vi "client handle page request.vi"(4 "error in (no error)":errorcluster, 7 "Client IP (\"\")":string) -> (0 "error out":errorcluster, 3 "Template Keys":T1)   [LabVIEW 2011]
uses:
  Addons/internet/utils/keyedarr.llb/Keyed Array.ctl
  Addons/internet/utils/strutil.llb/Case Matching.ctl
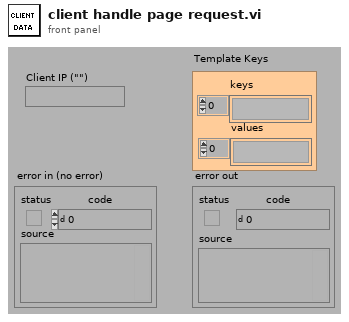
[diagram p1: front panel]
types:
  T1 = typedef "Keyed Array.ctl" = cluster{"keys":string[], "values":string[]}
  T2 = typedef "Case Matching.ctl" = enum16{"a != A", "a == A", "system"}
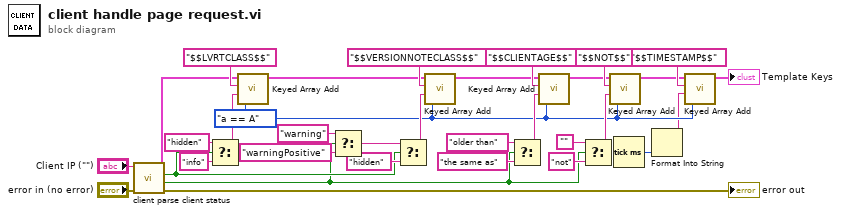
[diagram p0: block diagram]
diagram:
  w7 = Case_Matching."a == A" ("case matching (sensitive)")
  n1 = call "client parse client status.vi"("error in (no error)"="error in (no error)", "Client IP"="Client IP (\"\")") -> ("error out"=→"error out":errorcluster, "Update Needed?"=w2:bool, "Client Detected?"=w14:bool, "Client Status Keys"=w15:T1)  [unwired: 6 out]
  n2 = Select(t="hidden" ("Template (\"\")"), s=w14, f="info" ("Template (\"\")")) -> (s? t:f=w26:string)
  n3 = call "Keyed Array Add.vi"("case matching (sensitive)"=w7, "value"=w26, "key"="$$LVRTCLASS$$" ("Template (\"\")"), "array in"=w15) -> ("array out"=w31:T1)  [unwired: 3 out]
  n4 = Select(t="warning" ("Template (\"\")"), s=w2, f="warningPositive" ("Template (\"\")")) -> (s? t:f=w1:string)
  n5 = Select(t=w1, s=w14, f="hidden" ("Template (\"\")")) -> (s? t:f=w25:string)
  n6 = call "Keyed Array Add.vi"("case matching (sensitive)"=w7, "value"=w25, "key"="$$VERSIONNOTECLASS$$" ("Template (\"\")"), "array in"=w31) -> ("array out"=w29:T1)  [unwired: 3 out]
  n7 = Select(t="older than" ("Template (\"\")"), s=w2, f="the same as" ("Template (\"\")")) -> (s? t:f=w19:string)
  n8 = call "Keyed Array Add.vi"("case matching (sensitive)"=w7, "value"=w19, "key"="$$CLIENTAGE$$" ("Template (\"\")"), "array in"=w29) -> ("array out"=w27:T1)  [unwired: 3 out]
  n9 = Select(t="", s=w2, f="not" ("Template (\"\")")) -> (s? t:f=w16:string)
  n10 = call "Keyed Array Add.vi"("case matching (sensitive)"=w7, "value"=w16, "key"="$$NOT$$" ("Template (\"\")"), "array in"=w27) -> ("array out"=w9:T1)  [unwired: 3 out]
  n11 = Tick Count (ms)() -> (millisecond timer value=w6:u32)
  n12 = Format Into String(w6) -> (resulting string=w5:string)  [unwired: 3 in, 1 out]
  n13 = call "Keyed Array Add.vi"("case matching (sensitive)"=w7, "value"=w5, "key"="$$TIMESTAMP$$" ("Template (\"\")"), "array in"=w9) -> ("array out"=→"Template Keys":T1)  [unwired: 3 out]
